vi "ICM Recorder.vi"(11 "ICM Format":T2 {"Start Time" format="%<%H:%M:%S>t"; "Date" format="%<%Y/%m/%d>T"; "Version" format="%.1g"}) -> (10 "Stream File":path)   [LabVIEW 2018]
doc: "OSDS Recorder.vi\n\n This VI is used to record a time-stamped data stream so that it can be regenerated at a later time. It can also be used to load and view a previously recorded Stream file.\n\nOCC Streaming Data System Version 1.2.1\nMay, 2015 Original Code Consulting David Thomson\n www.originalcode.com\n\nOSDS is licensed under the Creative Commons Attribution-Share Alike 3.0 license (http://creativecommons.org/). Derivative and commercial works incorporating OSDS are allowed, as long as changes you make are made available to the community at large. Please submit improvements as well as new OSDS Format Files and OSDS Stream Files to support@originalcode.com"
uses:
  MICAS-X/Resources/OSDS/OSDS Subvis/OSDS Recorder State.ctl
  Instance           1 21Saved   OSDS Recorder .vi
  Instance           2 21Saved   OSDS Recorder .vi
  Instance           3 21Saved   OSDS Recorder .vi
  ICM Format.ctl
panel:
  out "Busy":bool
  out "Recorder State":T1
  out "Tab":enum32{"Setup", "Data"}(tab)
  in  "View":bool
  in  "Load Stream":bool
  in  "Load":bool
  in  "Record":bool
  in  "Return":bool
  in  "Display Style":enum16{"Normal", "Codes", "Password", "Hex"}(ring)
  out "Data":T3(array[cluster]) {"Time Stamp" format="%<%H:%M:%S%1u>t"}
  in  "Max Frame Time (ms)":i32=1000
  in  "Clear Error":bool
  in  "Stop Recording":bool
  out "Error":errorcluster
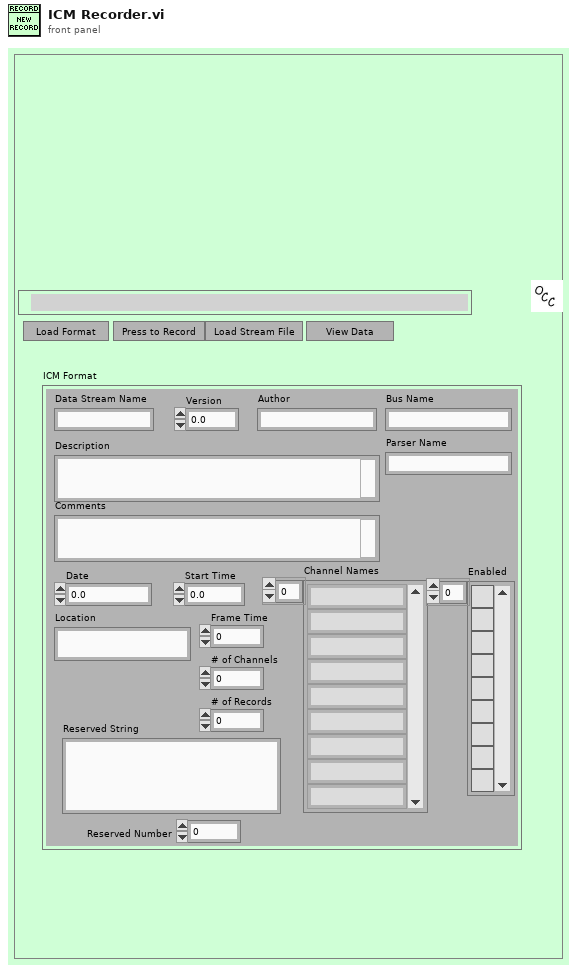
[diagram p1: front panel]
types:
  T1 = typedef "OSDS Recorder State.ctl" = enum16{"Initialize", "Wait", "Open File", "Open Port", "Write Query", "Read Char", "Write Char", "Update # Rec", "Open Stream", "Stop"}
  T2 = typedef "ICM Format.ctl" = cluster{"Data Stream Name":string, "Version":sgl, "Author":string, "Bus Name":string, "Parser Name":string, "Description":string, "Comments":string, "Location":string, "Frame Time":i32, "# of Channels":i32, "# of Records":i32, "Channel Names":string[], "Enabled":bool[], "Reserved String":string, "Reserved Number":dbl, "Date":dbl, "Start Time":dbl}
  T3 = cluster{"Time Stamp":dbl, "Length":i32, "Data":string}[]
  T4 = enum32{"invalid app kind", "Development System", "Run Time System", "Student Edition", "Embedded LabVIEW", "Evaluation", "Custom"}
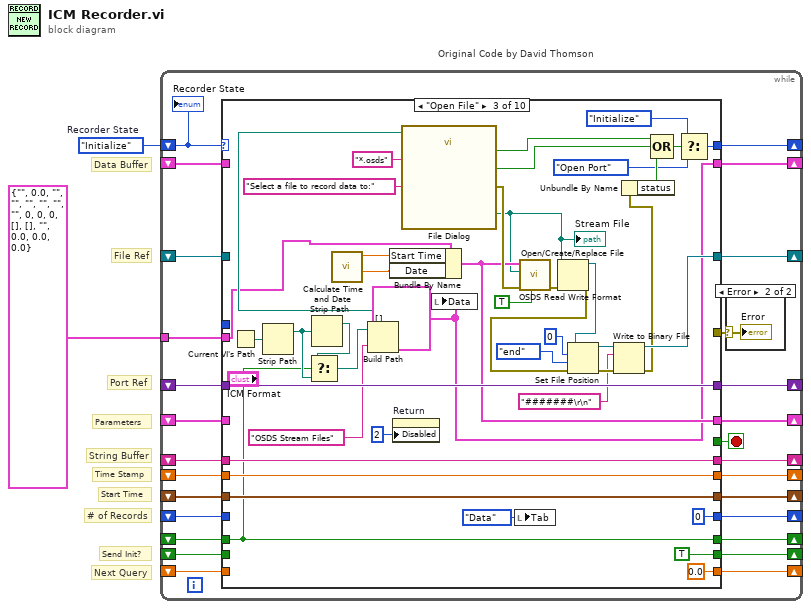
[diagram p0: block diagram]
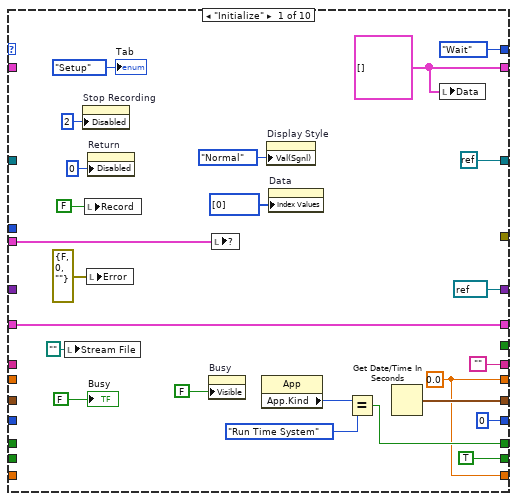
[diagram p3: hidden frame]
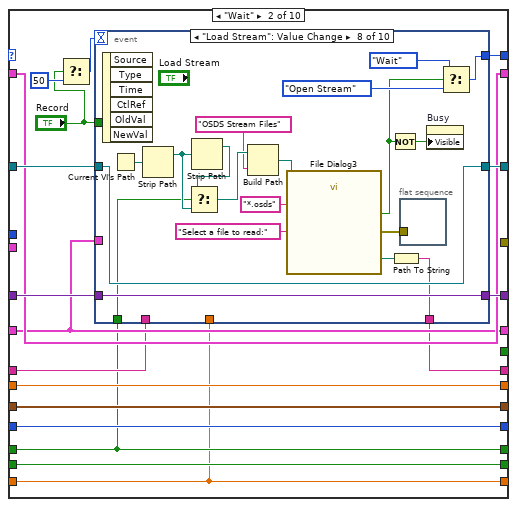
[diagram p4: hidden frame]
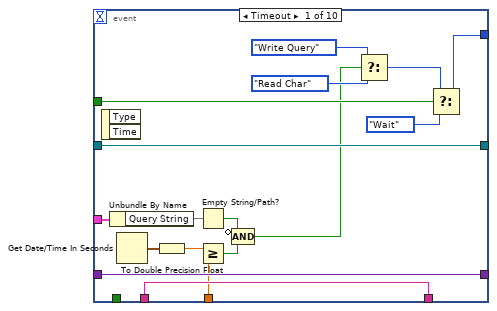
[diagram p5: hidden frame]
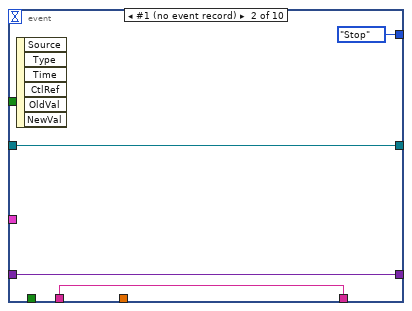
[diagram p6: hidden frame]
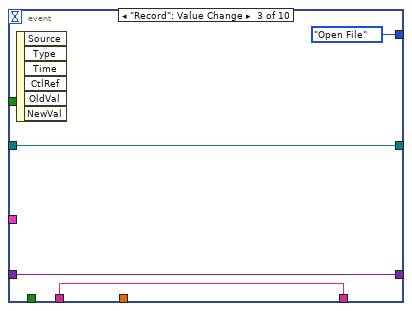
[diagram p7: hidden frame]
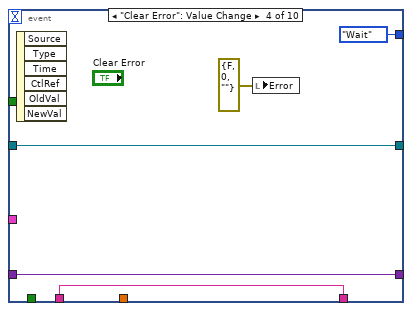
[diagram p8: hidden frame]
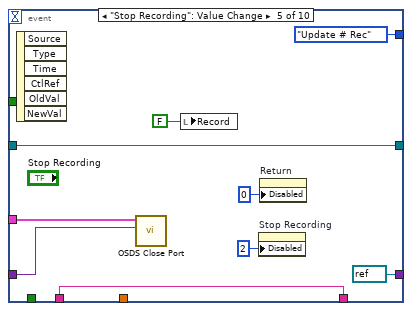
[diagram p9: hidden frame]
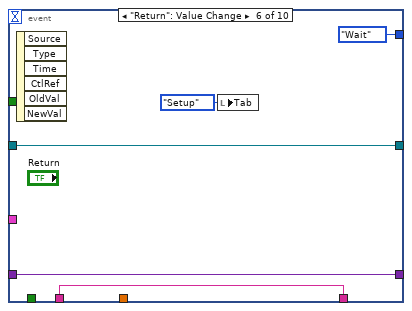
[diagram p10: hidden frame]
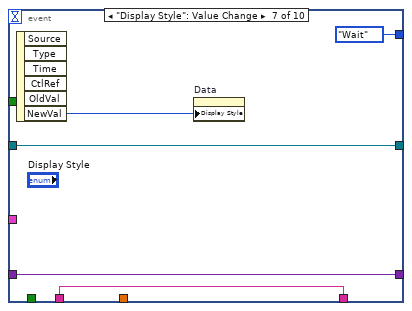
[diagram p11: hidden frame]
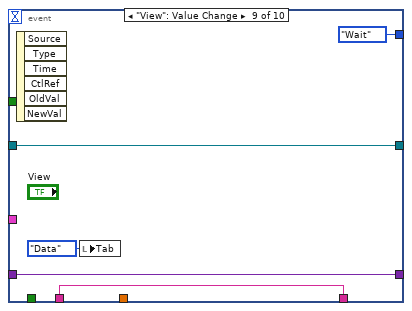
[diagram p12: hidden frame]
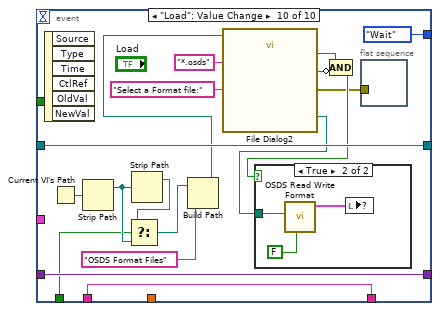
[diagram p13: hidden frame]
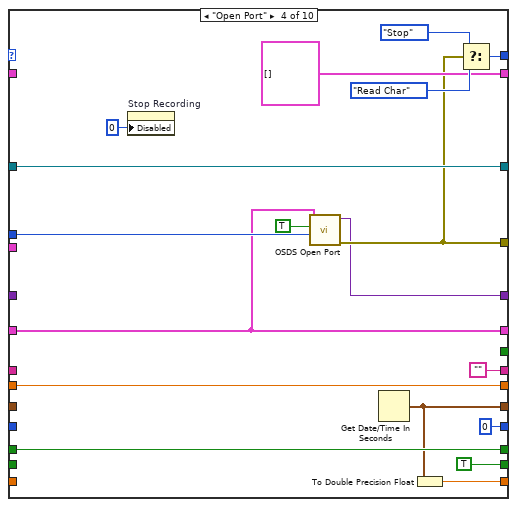
[diagram p15: hidden frame]
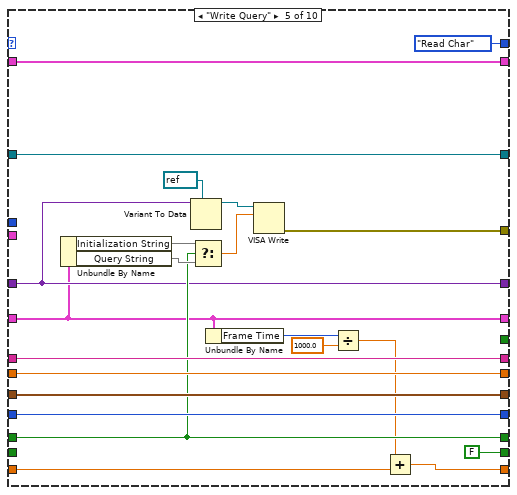
[diagram p16: hidden frame]
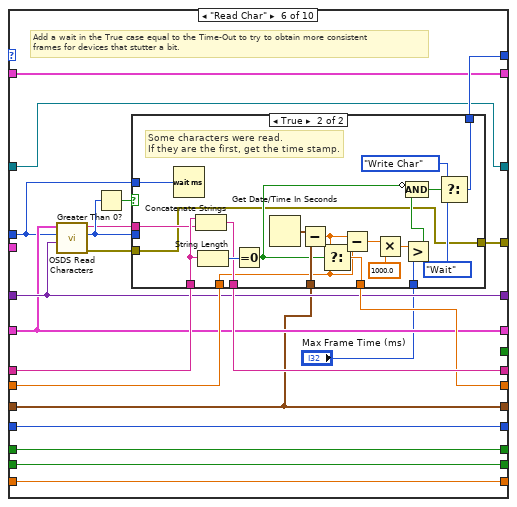
[diagram p17: hidden frame]
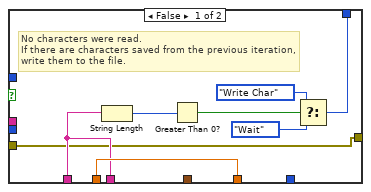
[diagram p18: hidden frame]
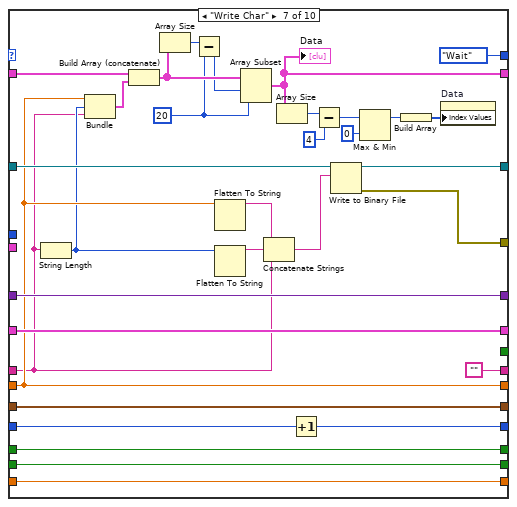
[diagram p19: hidden frame]
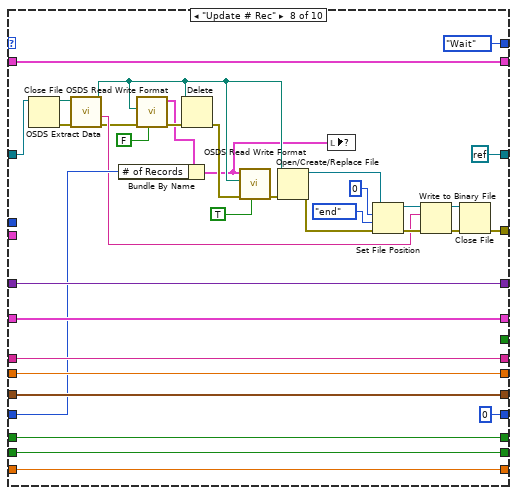
[diagram p20: hidden frame]
diagram:
  w2 = OSDS_Recorder_State."Initialize"  # Recorder State
  # "Next Query"
  # "Send Init?"
  # "# of Records"
  # "Data Buffer"
  # "Start Time"
  # "Time Stamp"
  # "String Buffer"
  # "Parameters"
  # "Port Ref"
  # "File Ref"
  n1 = while "Original Code by David Thomson" {
    shift-right: [w28] -> _
    shift-left: w2 -> [w29]
    shift-right: [w26] -> _
    shift-left: _ -> [w25]
    shift-right: [w24] -> _
    shift-left: _ -> [w23]
    shift-right: [w22] -> _
    shift-left: _ -> [w21]
    shift-right: [w16] -> _
    shift-left: _ -> [w17]
    shift-right: [w18] -> _
    shift-left: _ -> [w19]
    shift-right: [w15] -> _
    shift-left: _ -> [w14]
    shift-right: [w12] -> _
    shift-left: _ -> [w13]
    shift-right: [w11] -> _
    shift-left: _ -> [w10]
    tunnel: T2 {"Data Stream Name"="", "Version"=0.0, "Author"="", "Bus Name"="", "Parser Name"="", "Description"="", "Comments"="", "Location"="", "Frame Time"=0, "# of Channels"=0, "# of Records"=0, "Channel Names"=[], "Enabled"=[], "Reserved String"="", "Reserved Number"=0.0, "Date"=0.0, "Start Time"=0.0} ("OSDS Format") -> [w9]
    shift-right: [w8] -> _
    shift-left: _ -> [w7]
    shift-right: [w6] -> _
    shift-left: _ -> [w5]
    shift-right: [w3] -> _
    shift-left: _ -> [w4]
    stop <- w27 stop-if-true
    n2 = case shown="\"Open File\"" w29 {
      tunnel: [OSDS_Recorder_State."Wait" ("Recorder State") w72 w203 w226 OSDS_Recorder_State."Read Char" ("Recorder State") w268 OSDS_Recorder_State."Wait" ("Recorder State") OSDS_Recorder_State."Wait" ("Recorder State") OSDS_Recorder_State."Wait" ("Recorder State") OSDS_Recorder_State."Stop" ("Recorder State")] -> w28
      tunnel: [_ _ _ _ _ _ _ _ _ TRUE] -> w27
      tunnel: [refnum<k0> refnum w71 w189 w227 w248 w256 w326 refnum<k0> refnum w388 refnum<k0> refnum] -> w26
      tunnel: w25 -> [_ w70 _ w227 w248 w256 w327 w359 w388 w408]
      tunnel: [w51 w61 w186 w212 w231 w260 w331 w363 w386 w399] -> w24
      tunnel: w23 -> [w51 w61 _ w212 w231 w260 w331 w363 w386 w399]
      tunnel: [refnum<visa-resource-name> refnum ("VISA resource name out") w66 w198 w218 w238 w261 w330 w364 w387 refnum<visa-resource-name> refnum ("VISA resource name out")] -> w22
      tunnel: w21 -> [_ w67 w198 _ w238 w261 w330 w364 w387 w398]
      tunnel: [_ _ _ w219 w235 w266 w325 w344 w371 _] -> w20
      tunnel: w19 -> [_ w58 w197 _ w243 w269 w318 w362 w382 _]
      tunnel: ["" w59 w197 "" w243 w265 "" w362 w382 ""] -> w18
      tunnel: w17 -> [_ w65 w196 w222 w244 w267 w320 w361 w385 w403]
      tunnel: [w31 w65 w196 w222 w244 w264 w320 w361 w385 w403] -> w16
      tunnel: [w48 w64 w191 w213 w245 w250 w324 w360 w384 w402] -> w15
      tunnel: w14 -> [_ w64 w191 _ w245 w250 w324 w360 w384 w402]
      tunnel: w13 -> [_ w63 _ _ w249 w263 w315 w365 _ w401]
      tunnel: [w40 w63 w181 cluster{dbl, i32, string}[] [] w249 w263 w313 w365 w378 w401] -> w12
      tunnel: [0 w62 0 0 w246 w262 w316 0 w379 0] -> w11
      tunnel: w10 -> [_ w62 _ _ w246 w262 w317 w355 _ _]
      tunnel: _ -> [_ _ _ w217 _ w255 _ _ _ _]
      tunnel: w9 -> [w41 _ w167 _ _ _ _ _ _ _]
      tunnel: [w33 w57 w170 w215 w240 w254 w302 w334 w369 w392] -> w8
      tunnel: w7 -> [_ w57 w170 w215 w240 w254 w302 w334 w369 w392]
      tunnel: [TRUE ("Busy") w56 TRUE ("Busy") TRUE ("Busy") FALSE ("Busy") w253 w301 w333 w368 w391] -> w6
      tunnel: w5 -> [_ w56 _ _ _ w253 w301 w333 w368 w391]
      tunnel: [w31 w55 0.0 w211 w228 w252 w300 w332 w367 w390] -> w3
      tunnel: w4 -> [_ w55 _ _ w229 w252 w300 w332 w367 w390]
      frame "Initialize" {
        w40 = cluster{dbl, i32, string}[] []
        w31 = 0.0
        n3 = local write "Stream File"(path "") -> ()
        n4 = property on="Stop Recording" class="Bool"("Disabled"=u8 2) -> ()  [unwired: 2 in, 2 out]
        n5 = local write "Record"(FALSE ("Record")) -> ()
        n6 = local write "Error"(errorcluster {"status"=FALSE, "code"=0, "source"=""} ("Error")) -> ()
        n7 = property on="Return" class="Bool"("Disabled"=u8 0) -> ()  [unwired: 2 in, 2 out]
        n8 = property on="Busy" class="Bool (strict)"("Visible"=FALSE) -> ()  [unwired: 2 in, 2 out]
        n9 = local write item#-1(w41) -> ()
        n10 = property class="App"() -> ("App.Kind"=w35:T4)  [unwired: 2 in, 2 out]
        n11 = property on="Display Style" class="Enum (strict)"("Val(Sgnl)"=enum16{"Normal", "Codes", "Password", "Hex"}."Normal" ("Value (Signaling)")) -> ()  [unwired: 2 in, 2 out]
        n12 = property on="Data" class="Arr (strict)"("Index Values"=u32[] [0]) -> ()  [unwired: 2 in, 2 out]
        n13 = Equal?(x=w35, y=T4."Run Time System") -> (x = y?=w33:bool)
        n14 = Get Date/Time In Seconds() -> (seconds since 1Jan1904=w48:timestamp)
        n15 = local write "Data"(w40) -> ()
        "Tab" <- enum32{"Setup", "Data"}."Setup" ("Tab")
        "Busy" <- FALSE ("Busy")
      }
      frame "Wait" {
        n16 = Select(s="Record", f=50) -> (s? t:f=w69:i32)  [unwired: 1 in]
        n17 = event shown="[7] \"Load Stream\": Value Change" {
          selector: _ -> [_ _ _ _ _ _ _ _ _ _]
          dyn-events: _ -> [_ _ _ _ _ _ _ _ _ _]
          timeout: w69 -> [_ _ _ _ _ _ _ _ _ _]
          tunnel: [w89 OSDS_Recorder_State."Stop" ("Recorder State") OSDS_Recorder_State."Open File" ("Recorder State") OSDS_Recorder_State."Wait" ("Recorder State") OSDS_Recorder_State."Update # Rec" ("Recorder State") OSDS_Recorder_State."Wait" ("Recorder State") OSDS_Recorder_State."Wait" ("Recorder State") w137 OSDS_Recorder_State."Wait" ("Recorder State") OSDS_Recorder_State."Wait" ("Recorder State")] -> w72
          tunnel: [w87 w92 w96 w102 w110 w114 w119 w134 w145 w163] -> w71
          tunnel: w70 -> [w87 w92 w96 w102 w110 w114 w119 w134 w145 w163]
          tunnel: "Record" -> [w86 _ _ _ _ _ _ _ _ _]
          tunnel: w67 -> [w85 w91 w95 w99 w107 w113 w118 w140 w143 w161]
          tunnel: [w85 w91 w95 w99 refnum<visa-resource-name> refnum ("VISA resource name out") w113 w118 w140 w143 w161] -> w66
          tunnel: w61 -> [w83 _ _ _ w108 _ _ _ _ _]
          tunnel: [w84 w90 w94 w98 w104 w112 w117 w132 w141 w154] -> w59
          tunnel: w58 -> [w84 w90 w94 w98 w104 w112 w117 _ w141 w154]
          tunnel: w57 -> [_ _ _ _ _ _ _ w124 _ w147]
          tunnel: w55 -> [w81 _ _ _ _ _ _ _ _ _]
          event Timeout {
            n18 = event-data() -> ()  [unwired: 1 in, 2 out]
            n19 = Unbundle By Name(w83) -> ("Query String"=w82)
            n20 = Get Date/Time In Seconds() -> (seconds since 1Jan1904=w80:timestamp)
            n21 = To Double Precision Float(number=w80) -> (double precision float=w79:dbl)
            n22 = Empty String/Path?(string/path=w82) -> (empty?=w75:bool)
            n23 = Greater Or Equal?(x=w79, y=w81) -> (x >= y?=w74:bool)
            n24 = Compound Arithmetic op=AND(invert w75, w74) -> (w73:bool)
            n25 = Select(t=OSDS_Recorder_State."Write Query" ("Recorder State"), s=w73, f=OSDS_Recorder_State."Read Char" ("Recorder State")) -> (s? t:f=w76:T1)
            n26 = Select(t=w76, s=w86, f=OSDS_Recorder_State."Wait" ("Recorder State")) -> (s? t:f=w89:T1)
          }
          event #1 (no event record) {
            n27 = event-data() -> ()  [unwired: 1 in, 6 out]
          }
          event "Record": Value Change {
            n28 = event-data() -> ()  [unwired: 1 in, 6 out]
          }
          event "Clear Error": Value Change {
            n29 = event-data() -> ()  [unwired: 1 in, 6 out]
            n30 = local write "Error"(errorcluster {"status"=FALSE, "code"=0, "source"=""} ("Error")) -> ()
          }
          event "Stop Recording": Value Change {
            n31 = event-data() -> ()  [unwired: 1 in, 6 out]
            n32 = call "OSDS Close Port.vi"("Handle In"=w107, "OSDS Format"=w108) -> ()  [unwired: 9 in, 1 out]
            n33 = local write "Record"(FALSE ("Record")) -> ()
            n34 = property on="Stop Recording" class="Bool"("Disabled"=u8 2) -> ()  [unwired: 2 in, 2 out]
            n35 = property on="Return" class="Bool"("Disabled"=u8 0) -> ()  [unwired: 2 in, 2 out]
          }
          event "Return": Value Change {
            n36 = event-data() -> ()  [unwired: 1 in, 6 out]
            n37 = local write "Tab"(enum32{"Setup", "Data"}."Setup" ("Tab")) -> ()
          }
          event "Display Style": Value Change {
            n38 = event-data() -> ("NewVal"=w121:enum16{"Normal", "Codes", "Password", "Hex"})  [unwired: 1 in, 5 out]
            n39 = property on="Data" class="Str"("Display Style"=w121) -> ()  [unwired: 2 in, 2 out]
          }
          event "Load Stream": Value Change {
            n40 = event-data() -> ()  [unwired: 1 in, 6 out]
            n41 = Current VI's Path() -> (path=w128:path)
            n42 = Strip Path(path=w128) -> (stripped path=w125:path)  [unwired: 1 out]
            n43 = Strip Path(path=w125) -> (stripped path=w127:path)  [unwired: 1 out]
            n44 = Select(t=w127, s=w124, f=w125) -> (s? t:f=w126:path)
            n45 = Build Path(base path=w126, name or relative path="OSDS Stream Files") -> (appended path=w122:path)
            n46 = call "File Dialog3"("start path"=w122, "prompt"="Select a file to read:", "pattern (all files)"="*.osds") -> ("selected path"=w133:path, "cancelled"=w131:bool, "error out"=w129:errorcluster)  [unwired: 9 in, 1 out]
            n47 = Not(x=w131) -> (.not. x?=w130:bool)
            n48 = Path To String(path=w133) -> (string=w132:string)
            n49 = flat-sequence {
              tunnel: w129 -> [_]
              frame #0 {
              }
            }
            n50 = property on="Busy" class="Bool (strict)"("Visible"=w130) -> ()  [unwired: 2 in, 2 out]
            n51 = Select(t=OSDS_Recorder_State."Wait" ("Recorder State"), s=w131, f=OSDS_Recorder_State."Open Stream" ("Recorder State")) -> (s? t:f=w137:T1)
          }
          event "View": Value Change {
            n52 = event-data() -> ()  [unwired: 1 in, 6 out]
            n53 = local write "Tab"(enum32{"Setup", "Data"}."Data" ("Tab")) -> ()
          }
          event "Load": Value Change {
            n54 = event-data() -> ()  [unwired: 1 in, 6 out]
            n55 = Current VI's Path() -> (path=w152:path)
            n56 = Strip Path(path=w152) -> (stripped path=w150:path)  [unwired: 1 out]
            n57 = Strip Path(path=w150) -> (stripped path=w151:path)  [unwired: 1 out]
            n58 = Select(t=w151, s=w147, f=w150) -> (s? t:f=w149:path)
            n59 = Build Path(base path=w149, name or relative path="OSDS Format Files") -> (appended path=w148:path)
            n60 = call "File Dialog2"("start path"=w148, "prompt"="Select a Format file:", "pattern (all files)"="*.osds") -> ("selected path"=w155:path, "exists"=w158:bool, "cancelled"=w157:bool, "error out"=w153:errorcluster)  [unwired: 9 in]
            n61 = Compound Arithmetic op=AND(w158, invert w157) -> (w156:bool)
            n62 = case shown="True" w156 {
              tunnel: w155 -> [_ w166]
              frame False {
              }
              frame True {
                n63 = call "OSDS Read Write Format.vi"("Read/Write (Read)"=FALSE, "Format File"=w166) -> ("ICM Format Out"=w164:T2)  [unwired: 8 in, 1 out]
                n64 = local write item#-1(w164) -> ()
              }
            }
            n65 = flat-sequence {
              tunnel: w153 -> [_]
              frame #0 {
              }
            }
          }
        }
      }
      frame "Open File" {
        w181 = cluster{dbl, i32, string}[] []
        n66 = Current VI's Path() -> (path=w176:path)
        n67 = Strip Path(path=w176) -> (stripped path=w172:path)  [unwired: 1 out]
        n68 = Strip Path(path=w172) -> (stripped path=w173:path)  [unwired: 1 out]
        n69 = Select(t=w173, s=w170, f=w172) -> (s? t:f=w171:path)
        n70 = call "Calculate Time and Date.vi"() -> ("Date"=w184:dbl, "Time"=w185:dbl)  [unwired: 10 in]
        n71 = Build Path(base path=w171, name or relative path="OSDS Stream Files") -> (appended path=w174:path)
        n72 = Bundle By Name(cluster=w167, "Start Time"=w185, "Date"=w184) -> (w186:T2)
        n73 = property on="Return" class="Bool"("Disabled"=u8 2) -> ()  [unwired: 2 in, 2 out]
        n74 = call "File Dialog"("start path"=w174, "prompt"="Select a file to record data to:", "pattern (all files)"="*.osds") -> ("selected path"=w178:path, "exists"=w207:bool, "cancelled"=w206:bool, "error out"=w201:errorcluster)  [unwired: 9 in]
        "Stream File" <- w178
        n75 = local write "Data"(w181) -> ()
        n76 = local write "Tab"(enum32{"Setup", "Data"}."Data" ("Tab")) -> ()
        n77 = call "OSDS Read Write Format.vi"("Read/Write (Read)"=TRUE, "error in (no error)"=w201, "Format File"=w178, "ICM Format In"=w186) -> ("error out"=w200:errorcluster)  [unwired: 6 in, 1 out]
        n78 = Open/Create/Replace File(file path (use dialog)=w178, error in=w200) -> (refnum out=w195:refnum<file>, error out=w194:errorcluster)  [unwired: 4 in, 1 out]
        n79 = Set File Position(offset (in bytes) (0)=i64 0, refnum=w195, from (0:start)=enum16{"start", "end", "current"}."end", error in=w194) -> (refnum out=w190:refnum<file>, error out=w188:errorcluster)
        n80 = Write to Binary File(file (use dialog)=w190, data="#######\r\n", error in=w188) -> (refnum out=w189:refnum<file>, error out=w183:errorcluster)  [unwired: 3 in, 1 out]
        n81 = Unbundle By Name(w183) -> ("status"=w202:bool)
        n82 = Compound Arithmetic op=OR(w207, w206, w202) -> (w205:bool)
        n83 = Select(t=OSDS_Recorder_State."Initialize" ("Recorder State"), s=w205, f=OSDS_Recorder_State."Open Port" ("Recorder State")) -> (s? t:f=w203:T1)
      }
      frame "Open Port" {
        n84 = property on="Stop Recording" class="Bool"("Disabled"=u8 0) -> ()  [unwired: 2 in, 2 out]
        n85 = call "OSDS Open Port.vi"("timeout (ms)"=w217, "Recorder?"=TRUE, "OSDS Format"=w212) -> ("error out"=w219:errorcluster, "Handle Out"=w218:variant)  [unwired: 7 in]
        n86 = Get Date/Time In Seconds() -> (seconds since 1Jan1904=w213:timestamp)
        n87 = To Double Precision Float(number=w213) -> (double precision float=w211:dbl)
        n88 = Select(t=OSDS_Recorder_State."Stop" ("Recorder State"), s=w219, f=OSDS_Recorder_State."Read Char" ("Recorder State")) -> (s? t:f=w226:T1)
      }
      frame "Write Query" {
        n89 = Unbundle By Name(w231) -> ("Initialization String"=w242, "Query String"=w241)
        n90 = Variant To Data(type=refnum<visa-resource-name> refnum ("VISA resource name"), Variant=w238) -> (data=w237:refnum<visa-resource-name>)  [unwired: 1 in, 1 out]
        n91 = Select(t=w242, s=w240, f=w241) -> (s? t:f=w236:dbl)
        n92 = Unbundle By Name(w231) -> ("Frame Time"=w233:i32)
        n93 = VISA Write(VISA resource name=w237, write buffer=w236) -> (error out=w235:errorcluster)  [unwired: 1 in, 2 out]
        n94 = Divide(x=w233, y=1000.0) -> (x/y=w230:dbl)
        n95 = Add(x=w230, y=w229) -> (x+y=w228:dbl)
      }
      frame "Read Char" {
        # "Add a wait in the True case equal to the Time-Out to try to obtain more consistent\nframes for devices that stutter a bit."
        n96 = call "OSDS Read Characters.vi"("Handle In"=w261, "Timeout (ms)"=w255, "OSDS Format"=w260) -> ("error out"=w257:errorcluster, "Bytes Read"=w259:i32, "Data Out"=w258:string)  [unwired: 5 in, 1 out]
        n97 = Greater Than 0?(x=w259) -> (x > 0?=w270:bool)
        n98 = case shown="True" w270 {
          tunnel: w259 -> [_ _]
          tunnel: w257 -> [w271 w280]
          tunnel: w269 -> [w272 w299]
          tunnel: w267 -> [w278 w286]
          tunnel: [w278 w297] -> w264
          tunnel: [w275 w292] -> w268
          tunnel: "Max Frame Time (ms)" -> [_ w293]
          tunnel: [w271 w280] -> w266
          tunnel: w250 -> [_ w289]
          tunnel: [w272 w288] -> w265
          tunnel: w258 -> [_ w281]
          tunnel: w255 -> [_ w279]
          frame False {
            # "No characters were read.\nIf there are characters saved from the previous iteration,\nwrite them to the file."
            n99 = String Length(string=w272) -> (length=w277:i32)
            n100 = Greater Than 0?(x=w277) -> (x > 0?=w276:bool)
            n101 = Select(t=OSDS_Recorder_State."Write Char" ("Recorder State"), s=w276, f=OSDS_Recorder_State."Wait" ("Recorder State")) -> (s? t:f=w275:T1)
          }
          frame True {
            # "Some characters were read.\nIf they are the first, get the time stamp."
            n102 = Wait (ms)(milliseconds to wait=w279) -> ()  [unwired: 1 out]
            n103 = Concatenate Strings(w299, w281) -> (w288:string)
            n104 = String Length(string=w299) -> (length=w298:i32)
            n105 = Equal To 0?(x=w298) -> (x = 0?=w282:bool)
            n106 = Get Date/Time In Seconds() -> (seconds since 1Jan1904=w296:timestamp)
            n107 = Subtract(x=w296, y=w289) -> (x-y=w287:dbl)
            n108 = Select(t=w287, s=w282, f=w286) -> (s? t:f=w297:dbl)
            n109 = Subtract(x=w287, y=w286) -> (x-y=w285:dbl)
            n110 = Multiply(x=w285, y=1000.0) -> (x*y=w294:dbl)
            n111 = Greater?(x=w294, y=w293) -> (0:w283:bool)
            n112 = Compound Arithmetic op=AND(invert w282, w283) -> (w284:bool)
            n113 = Select(t=OSDS_Recorder_State."Write Char" ("Recorder State"), s=w284, f=OSDS_Recorder_State."Wait" ("Recorder State")) -> (s? t:f=w292:T1)
          }
        }
      }
      frame "Write Char" {
        w304 = 20 ("length")
        n114 = String Length(string=w318) -> (length=w319:i32)
        n115 = Bundle(w320, w319, w318) -> (w314:cluster{dbl, i32, string})  [unwired: 1 in]
        n116 = Build Array (concatenate)(w315, w314) -> (w306:T3)
        n117 = Array Size(array=w306) -> (size(s)=w305:i32)
        n118 = Subtract(x=w305, y=w304) -> (x-y=w303:i32)
        n119 = Flatten To String(anything=w320) -> (data string=w323:string)  [unwired: 3 in, 2 out]
        n120 = Flatten To String(anything=w319) -> (data string=w322:string)  [unwired: 3 in, 2 out]
        n121 = Array Subset(array=w306, index=w303, length=w304) -> (w313:T3)
        "Data" <- w313
        n122 = Concatenate Strings(w323, w322, w318) -> (w321:string)
        n123 = Array Size(array=w313) -> (size(s)=w312:i32)
        n124 = Increment(x=w317) -> (x+1=w316:i32)
        n125 = Subtract(x=w312, y=4) -> (x-y=w310:i32)
        n126 = Write to Binary File(file (use dialog)=w327, data=w321) -> (refnum out=w326:refnum<file>, error out=w325:errorcluster)  [unwired: 4 in, 1 out]
        n127 = Max & Min(x=w310, y=0) -> (max(x,y)=w309:i32)  [unwired: 1 out]
        n128 = Build Array(w309) -> (w308:i32[])
        n129 = property on="Data" class="Arr (strict)"("Index Values"=w308) -> ()  [unwired: 2 in, 2 out]
      }
      frame "Update # Rec" {
        n130 = Close File(refnum=w359) -> (path=w341:path, error out=w340:errorcluster)  [unwired: 1 in]
        n131 = call "OSDS Extract Data.vi"("error in (no error)"=w340, "Stream File"=w341) -> ("error out"=w338:errorcluster, "Stream Data with Separator"=w339:string, "Stream File Out"=w336:path)  [unwired: 6 in, 1 out]
        n132 = call "OSDS Read Write Format.vi"("Read/Write (Read)"=FALSE, "error in (no error)"=w338, "Format File"=w336) -> ("error out"=w354:errorcluster, "ICM Format Out"=w337:T2)  [unwired: 7 in]
        n133 = Bundle By Name(cluster=w337, "# of Records"=w355) -> (w335:T2)
        n134 = Delete(path (use dialog)=w336, error in=w354) -> (error out=w352:errorcluster)  [unwired: 3 in, 2 out]
        n135 = call "OSDS Read Write Format.vi"("Read/Write (Read)"=TRUE, "error in (no error)"=w352, "Format File"=w336, "ICM Format In"=w335) -> ("error out"=w351:errorcluster)  [unwired: 6 in, 1 out]
        n136 = Open/Create/Replace File(file path (use dialog)=w336, error in=w351) -> (refnum out=w345:refnum<file>, error out=w346:errorcluster)  [unwired: 4 in, 1 out]
        n137 = local write item#-1(w335) -> ()
        n138 = Set File Position(offset (in bytes) (0)=i64 0, refnum=w345, from (0:start)=enum16{"start", "end", "current"}."end", error in=w346) -> (refnum out=w348:refnum<file>, error out=w347:errorcluster)
        n139 = Write to Binary File(file (use dialog)=w348, data=w339, error in=w347) -> (refnum out=w342:refnum<file>, error out=w343:errorcluster)  [unwired: 3 in, 1 out]
        n140 = Close File(refnum=w342, error in=w343) -> (error out=w344:errorcluster)  [unwired: 1 out]
      }
      frame "Open Stream" {
        n141 = String To Path(string=w382) -> (path=w374:path)
        n142 = call "OSDS Read Write Format.vi"("Read/Write (Read)"=FALSE, "Format File"=w374) -> ("error out"=w377:errorcluster, "ICM Format Out"=w376:T2)  [unwired: 8 in]
        n143 = local write "Tab"(enum32{"Setup", "Data"}."Data" ("Tab")) -> ()
        n144 = property on="Data" class="Arr (strict)"("Index Values"=u32[] [0]) -> ()  [unwired: 2 in, 2 out]
        n145 = local write item#-1(w376) -> ()
        n146 = call "OSDS Extract Data.vi"("error in (no error)"=w377, "Stream File"=w374) -> ("error out"=w371:errorcluster, "Stream Data"=w381:string)  [unwired: 6 in, 2 out]
        n147 = local write "Error"(errorcluster {"status"=FALSE, "code"=0, "source"=""} ("Error")) -> ()
        n148 = local write "Stream File"(w374) -> ()
        n149 = call "OSDS Calculate Records.vi"("Assemble?"=TRUE, "Stream Data"=w381) -> ("Data"=w378:T3, "# of Records"=w379:i32)  [unwired: 8 in]
        n150 = local write "Data"(w378) -> ()
        n151 = property on="Busy" class="Bool (strict)"(error in=w371, "Visible"=FALSE) -> ()  [unwired: 1 in, 2 out]
      }
      frame "Stop" {
        n152 = property on="Return" class="Bool"("Disabled"=u8 0) -> ()  [unwired: 2 in, 2 out]
        n153 = Close File(refnum=w408) -> (error out=w394:errorcluster)  [unwired: 1 in, 1 out]
        n154 = local write "Record"(FALSE ("Record")) -> ()
        n155 = call "OSDS Close Port.vi"("Handle In"=w398, "OSDS Format"=w399) -> ("error out"=w393:errorcluster)  [unwired: 9 in]
        n156 = case shown="True" w392 {
          tunnel: w394 -> [_ _]
          tunnel: w393 -> [_ _]
          frame False {
          }
          frame True {
            n157 = property class="VI"("Front Panel.Open"=FALSE ("Front Panel Window:Open")) -> ()  [unwired: 2 in, 2 out]
          }
        }
        n158 = property on="Stop Recording" class="Bool"("Disabled"=u8 2) -> ()  [unwired: 2 in, 2 out]
      }
    }
    n159 = case shown="Error" w20 {
      selector: w20 -> [_ w30]
      frame No Error {
      }
      frame Error {
        "Error" <- w30
      }
    }
    "Recorder State" <- w29
  }
